vi "TL behavior get unstuck.vi"(1 "Behavior\nVelocity":dbl, 2 "Activate?":bool=TRUE, 3 "Sensor":T1=[{"Name"="bow", "Angle"=20.0, "Distance"=0.0}, {"Name"="pbow", "Angle"=60.0, "Distance"=0.0}, {"Name"="port", "Angle"=0.0, "Distance"=0.0}, {"Name"="sbow", "Angle"=60.0, "Distance"=0.0}, {"Name"="starboard", "Angle"=0.0, "Distance"=0.0}]) -> (0 "Unstuck Array":dbl[](array[numeric]))   [LabVIEW 2014]
uses:
  sensorsSTD.ctl
panel:
  out "Waveform Graph":cluster{dbl, dbl, dbl[]}(graph)
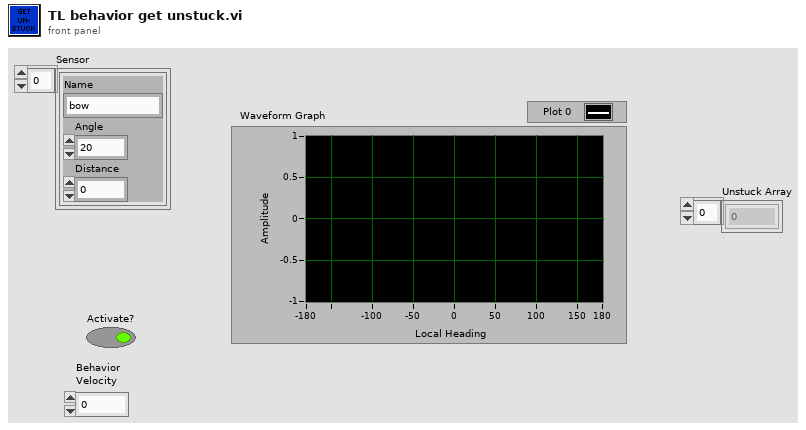
[diagram p1: front panel]
types:
  T1 = typedef "sensorsSTD.ctl" = cluster{"Name":string, "Angle":dbl, "Distance":dbl}[]
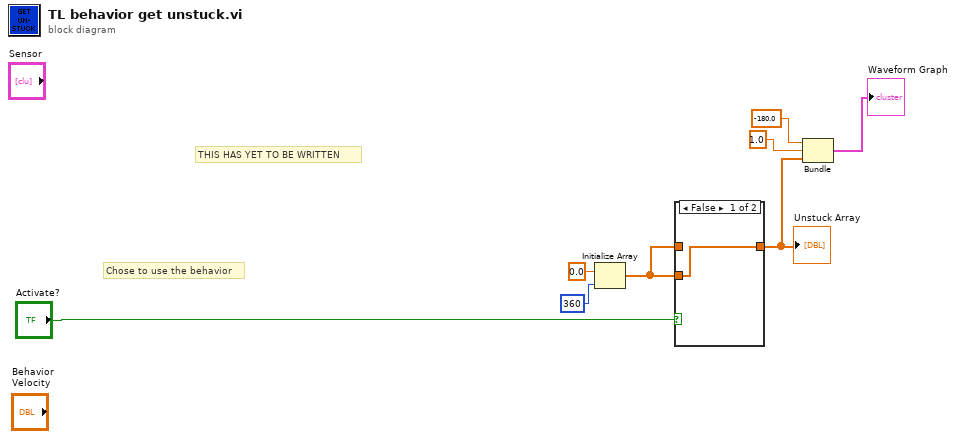
[diagram p0: block diagram]
diagram:
  # "THIS HAS YET TO BE WRITTEN"
  # "Chose to use the behavior"
  n1 = Initialize Array(0.0 ("element"), 360 ("dimension size")) -> (w2:dbl[])
  n2 = case shown="False" "Activate?" {
    tunnel: w2 -> [w9 _]
    tunnel: w2 -> [_ w10]
    tunnel: [w9 w10] -> w1
    frame False {
    }
    frame True {
    }
  }
  "Unstuck Array" <- w1
  n3 = Bundle(-180.0, 1.0, w1) -> (→"Waveform Graph":cluster{dbl, dbl, dbl[]})  [unwired: 1 in]
